vi "get channels.vi"(8 "error in (no error)":errorcluster, 11 "action configuration in":refnum<class "action configuration.lvclass">) -> (0 "error out":errorcluster, 2 "action channels":refnum<class "TBM channel.lvclass">[](array[class]), 3 "action configuration out":refnum<class "action configuration.lvclass">)   [LabVIEW 2014, in "action configuration.lvclass"]
doc: "Returns the list of channels this instance of the Action is configured to interact with."
uses:
  action configuration.lvclass
  <vilib>/NI/Tag Bus Module Framework/channel/TBM channel.lvclass
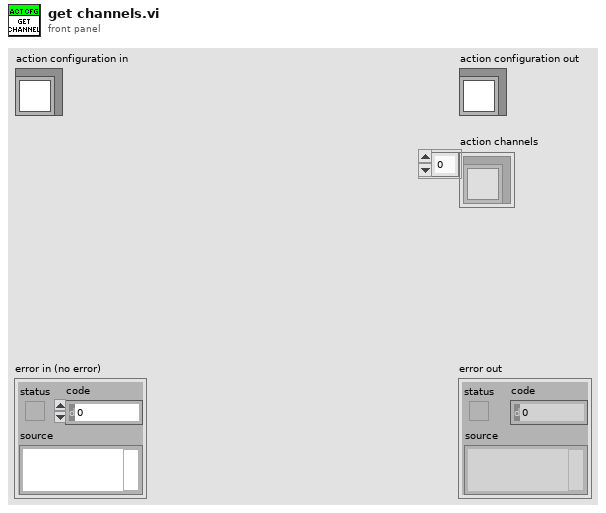
[diagram p1: front panel]
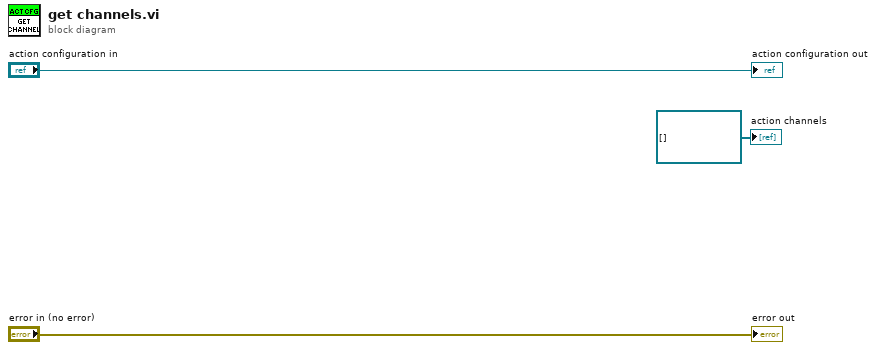
[diagram p0: block diagram]
diagram:
  "error out" <- "error in (no error)"
  "action configuration out" <- "action configuration in"
  "action channels" <- refnum<class "TBM channel.lvclass">[] [] ("action channels")
